vi "Script Msg Output Private Data.vi"(6 "Name Msg Output Refs.Private Data Cluster":refnum<vi>, 8 "error in":errorcluster, 9 "Name Msg Output Refs.Private Data Control":refnum<vi>, 10 "Msg Output Terminal Attributes":T1) -> (0 "error out":errorcluster)   [LabVIEW 2025, in "_Rescript.lvlib" / "_Rescript.lvclass"]
uses:
  _Rescript.lvclass
  Terminal Attributes.ctl
  Attributes.ctl
  <vilib>/Utility/miscctls.llb/LVPositionTypeDef.ctl
  _Rescript.lvclass/_Rescript.ctl
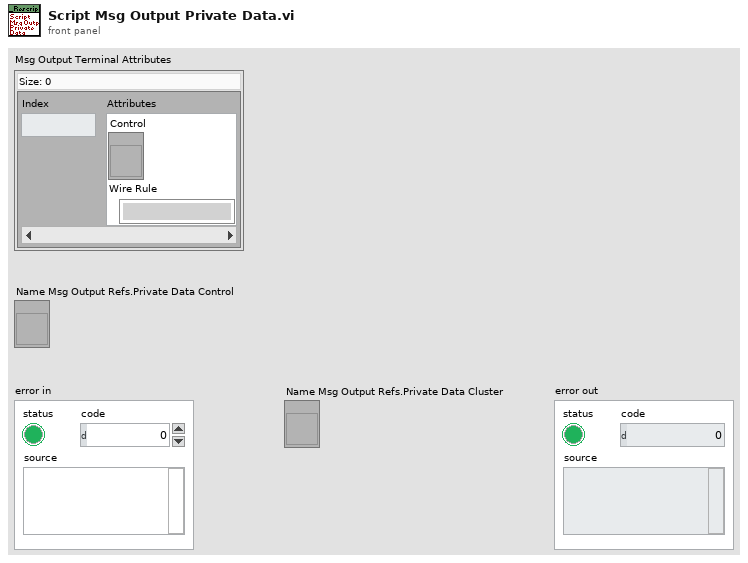
[diagram p1: front panel]
types:
  T1 = typedef "_Rescript.lvlib/_Rescript.lvclass/Terminal Attributes.ctl" = map{i32, T2}
  T2 = typedef "_Rescript.lvlib/_Rescript.lvclass/Attributes.ctl" = cluster{"Control":refnum<vi>, "Wire Rule":enum16{"Invalid Wire Rule", "Required", "Recommended", "Optional", "Dynamic Dispatch"}}
  T3 = typedef "LVPositionTypeDef.ctl" = cluster{"Left":i32, "Top":i32}
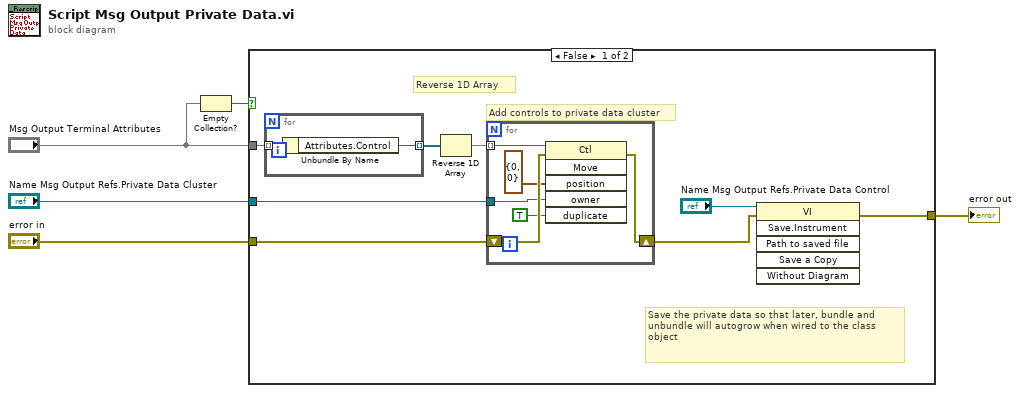
[diagram p0: block diagram]
diagram:
  n1 = Empty Collection?(1:"Msg Output Terminal Attributes") -> (0:w2:bool)
  n2 = case shown="False" w2 {
    tunnel: [w12 w22] -> w5
    tunnel: "error in" -> [w11 w22]
    tunnel: "Name Msg Output Refs.Private Data Cluster" -> [w9 _]
    tunnel: "Msg Output Terminal Attributes" -> [w6 _]
    frame False {
      # "Reverse 1D Array"
      # "Add controls to private data cluster"
      # "Save the private data so that later, bundle and unbundle will autogrow when wired to the class object"
      n3 = for {
        tunnel: w6 -> [w15] mode=indexing
        tunnel: [w14] -> w8 mode=indexing
        n4 = Unbundle By Name(w15) -> ("Attributes.Control"=w14:refnum<vi>)
      }
      n5 = Reverse 1D Array(array=w8) -> (reversed array=w7:refnum<vi>[])
      n6 = for {
        tunnel: w9 -> [w20]
        shift-right: [w19] -> w13
        shift-left: w11 -> [w21]
        tunnel: w7 -> [w18] mode=indexing
        n7 = invoke class="Ctl" method="Move"(reference=w18, error in=w21, "position"=T3 {"Left"=0, "Top"=0}, "owner"=w20, "duplicate"=TRUE ("Duplicate? (F)")) -> (error out=w19:errorcluster)  [unwired: 1 in, 5 out]
      }
      n8 = invoke class="VI" method="Save.Instrument"(reference="Name Msg Output Refs.Private Data Control", error in=w13) -> (error out=w12:errorcluster)  [unwired: 4 in, 5 out]
    }
    frame True {
    }
  }
  "error out" <- w5
